vi "writeToXML.vi"(8 "error in (no error)":errorcluster, 10 "ClassLabel":string, 11 "MccDisable in":refnum<class "MccDisable.lvclass">) -> (0 "error out":errorcluster, 2 "XMLout":string, 3 "MccDisable out":refnum<class "MccDisable.lvclass">)   [LabVIEW 2022 SP3, in "TCSDataDefinitions.lvlib" / "TCSMountControlCommand.lvlib" / "CommandsForAllAxes.lvlib" / "MccDisable.lvclass"]
uses:
  MccDisable.lvclass
  CommandsForAllAxes.lvclass
  <userlib>/Common/XML/XMLGenerator/XMLGenerator.lvclass
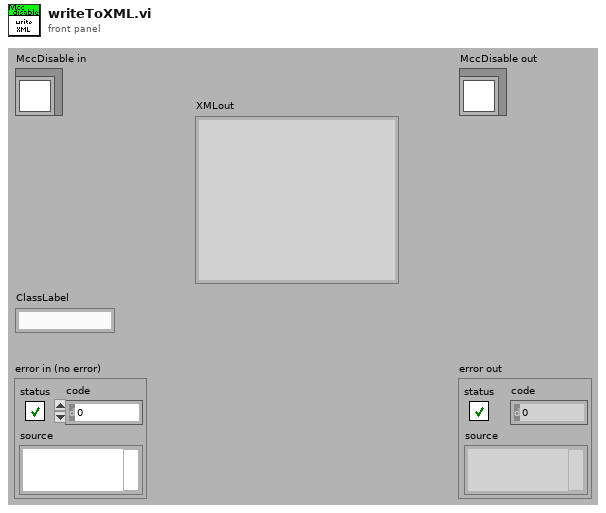
[diagram p1: front panel]
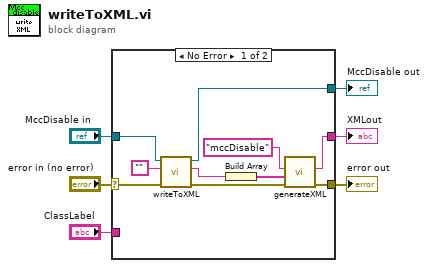
[diagram p0: block diagram]
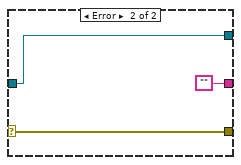
[diagram p2: hidden frame]
diagram:
  n1 = case shown="No Error" "error in (no error)" {
    selector: "error in (no error)" -> [w14 w19]
    tunnel: [w9 w19] -> w5
    tunnel: [w15 w18] -> w3
    tunnel: "MccDisable in" -> [w16 w18]
    tunnel: [w7 ""] -> w2
    tunnel: "ClassLabel" -> [_ _]
    frame No Error {
      n2 = call-parent "writeToXML.vi"("error in (no error)"=w14, "ClassLabel"="", "CommandsForAllAxes in"=w16) -> ("error out"=w10:errorcluster, "XMLout"=w12:string, "CommandsForAllAxes out"=w15:refnum<class "MccDisable.lvclass">)  [unwired: 6 in]
      n3 = Build Array(w12) -> (w13:string[])
      n4 = call <userlib>:"generateXML.vi"("error in"=w10, "childrenXML"=w13, "elementName"="mccDisable" ("Class Label")) -> ("error out"=w9:errorcluster, "XML out"=w7:string)  [unwired: 6 in, 1 out]
    }
    frame Error {
    }
  }
  "error out" <- w5
  "MccDisable out" <- w3
  "XMLout" <- w2
